vi "GetParam.vi"(8 "error in (no error)":errorcluster caption="entrée d'erreur (pas d'erreur)", 11 "OrdinalEncoder.lvclass":refnum<class "OrdinalEncoder.lvclass">) -> (0 "error out":errorcluster caption="sortie d'erreur", 2 "OrdinalEncoder":cluster{"dtype":string}={"dtype"="float"}, 3 "OrdinalEncoder.lvclass":refnum<class "OrdinalEncoder.lvclass">)   [LabVIEW 2020, in "OrdinalEncoder.lvclass"]
doc: "Get Parameters"
uses:
  OrdinalEncoder.lvclass
  OrdinalEncoder.lvclass/OrdinalEncoder.ctl
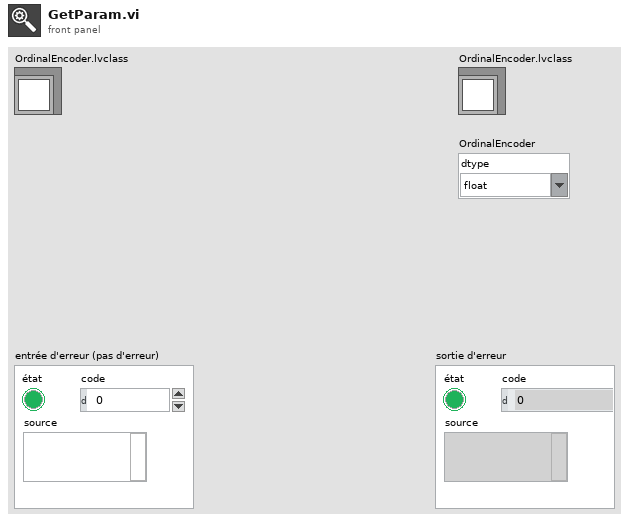
[diagram p1: front panel]
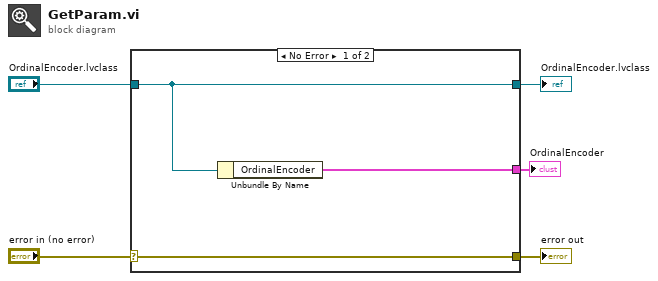
[diagram p0: block diagram]
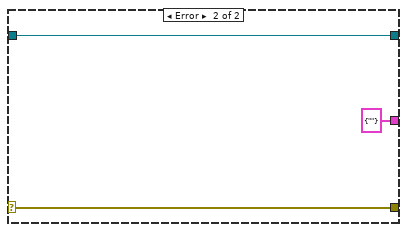
[diagram p2: hidden frame]
diagram:
  n1 = case shown="No Error" "error in (no error)" {
    selector: "error in (no error)" -> [w8 w10]
    tunnel: [w8 w10] -> w4
    tunnel: [w7 w11] -> w2
    tunnel: "OrdinalEncoder.lvclass" -> [w7 w11]
    tunnel: [w6 cluster{"dtype":string} {"dtype"=""} ("OrdinalEncoder")] -> w1
    frame No Error {
      n2 = Unbundle By Name(w7) -> ("OrdinalEncoder"=w6:cluster{"dtype":string})
    }
    frame Error {
    }
  }
  "error out" <- w4
  "OrdinalEncoder.lvclass" <- w2
  "OrdinalEncoder" <- w1
